vi "I2C_SDA_DAQ.vi"(1 "Tx_or_Rx?":bool, 3 "Tx_Data":bool) -> (0 "Rx_Data":bool)   [LabVIEW 2022 SP3]
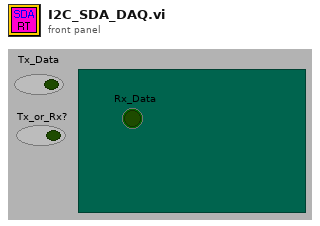
[diagram p1: front panel]
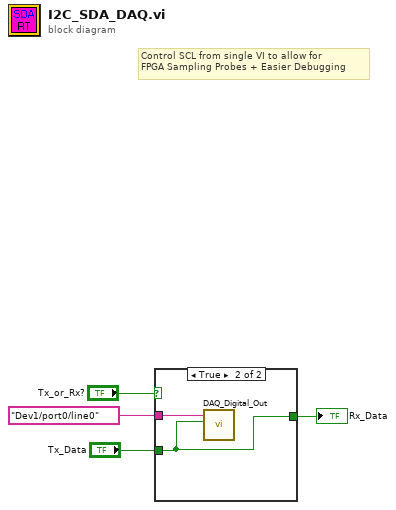
[diagram p0: block diagram]
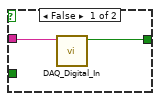
[diagram p2: hidden frame]
diagram:
  # "Control SCL from single VI to allow for \nFPGA Sampling Probes + Easier Debugging"
  n1 = case shown="True" "Tx_or_Rx?" {
    tunnel: "Dev1/port0/line0" ("Output Chanel") -> [w6 w8]
    tunnel: [w5 w7] -> w2
    tunnel: "Tx_Data" -> [_ w7]
    frame False {
      n2 = call "DAQ_Digital_In.vi"("Input Chanel"=w6) -> ("Read"=w5:bool)  [unwired: 9 in, 1 out]
    }
    frame True {
      n3 = call "DAQ_Digital_Out.vi"("Write"=w7, "Output Chanel"=w8) -> ()  [unwired: 9 in, 1 out]
    }
  }
  "Rx_Data" <- w2
